vi "helipadDataOrganiser.vi"(3 "Number of Heights":i32=4, 4 "Number of Files":i32=4, 5 "Method A (Left), Method B (Right)":bool, 6 "Data Path":string) -> (0 "Output Data":string[][](array[string]), 1 "Probe No":string, 2 "In Folder":string)   [LabVIEW 2018]
uses:
  <vilib>/Utility/file.llb/Read Delimited Spreadsheet (string).vi
panel:
  in  "Tab Control":enum32{"Pull Method A", "Pull Method B"}(tab)
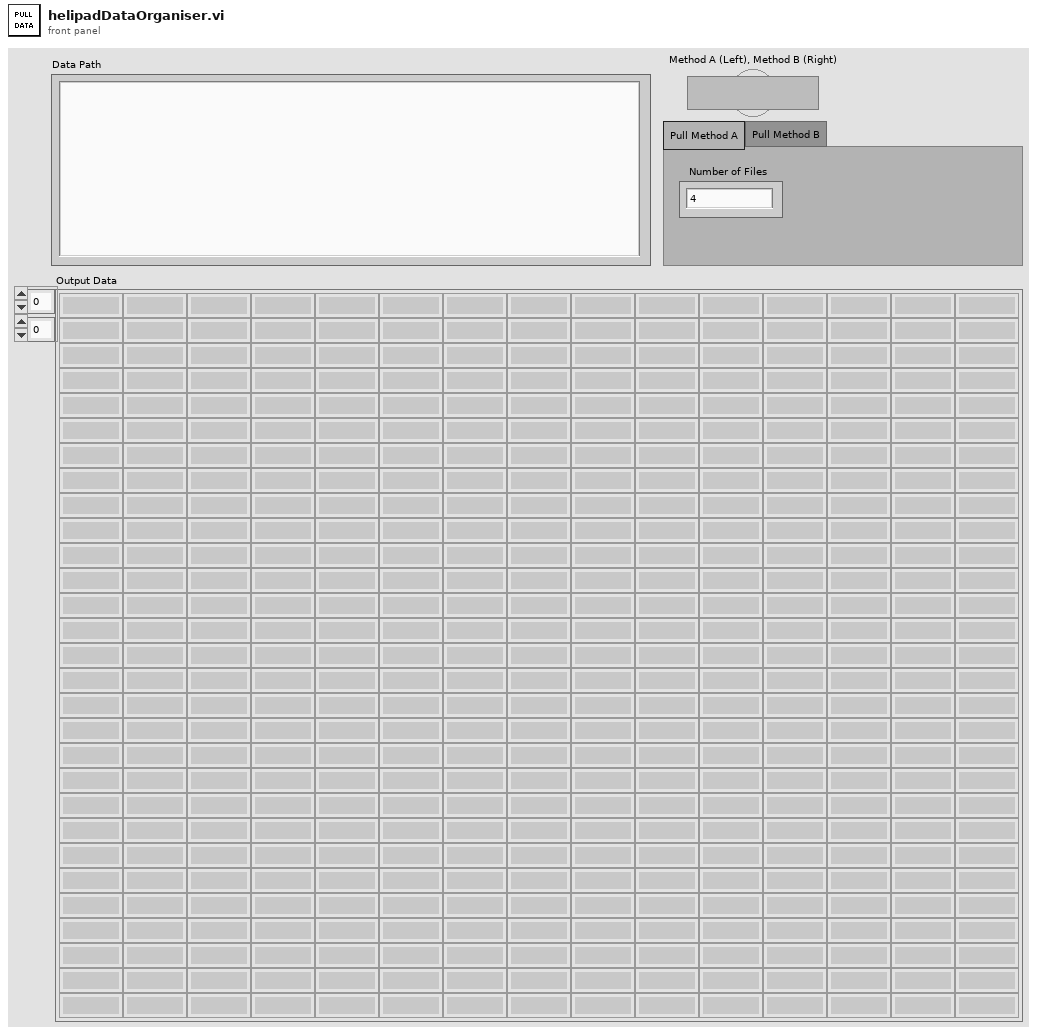
[diagram p1: front panel]
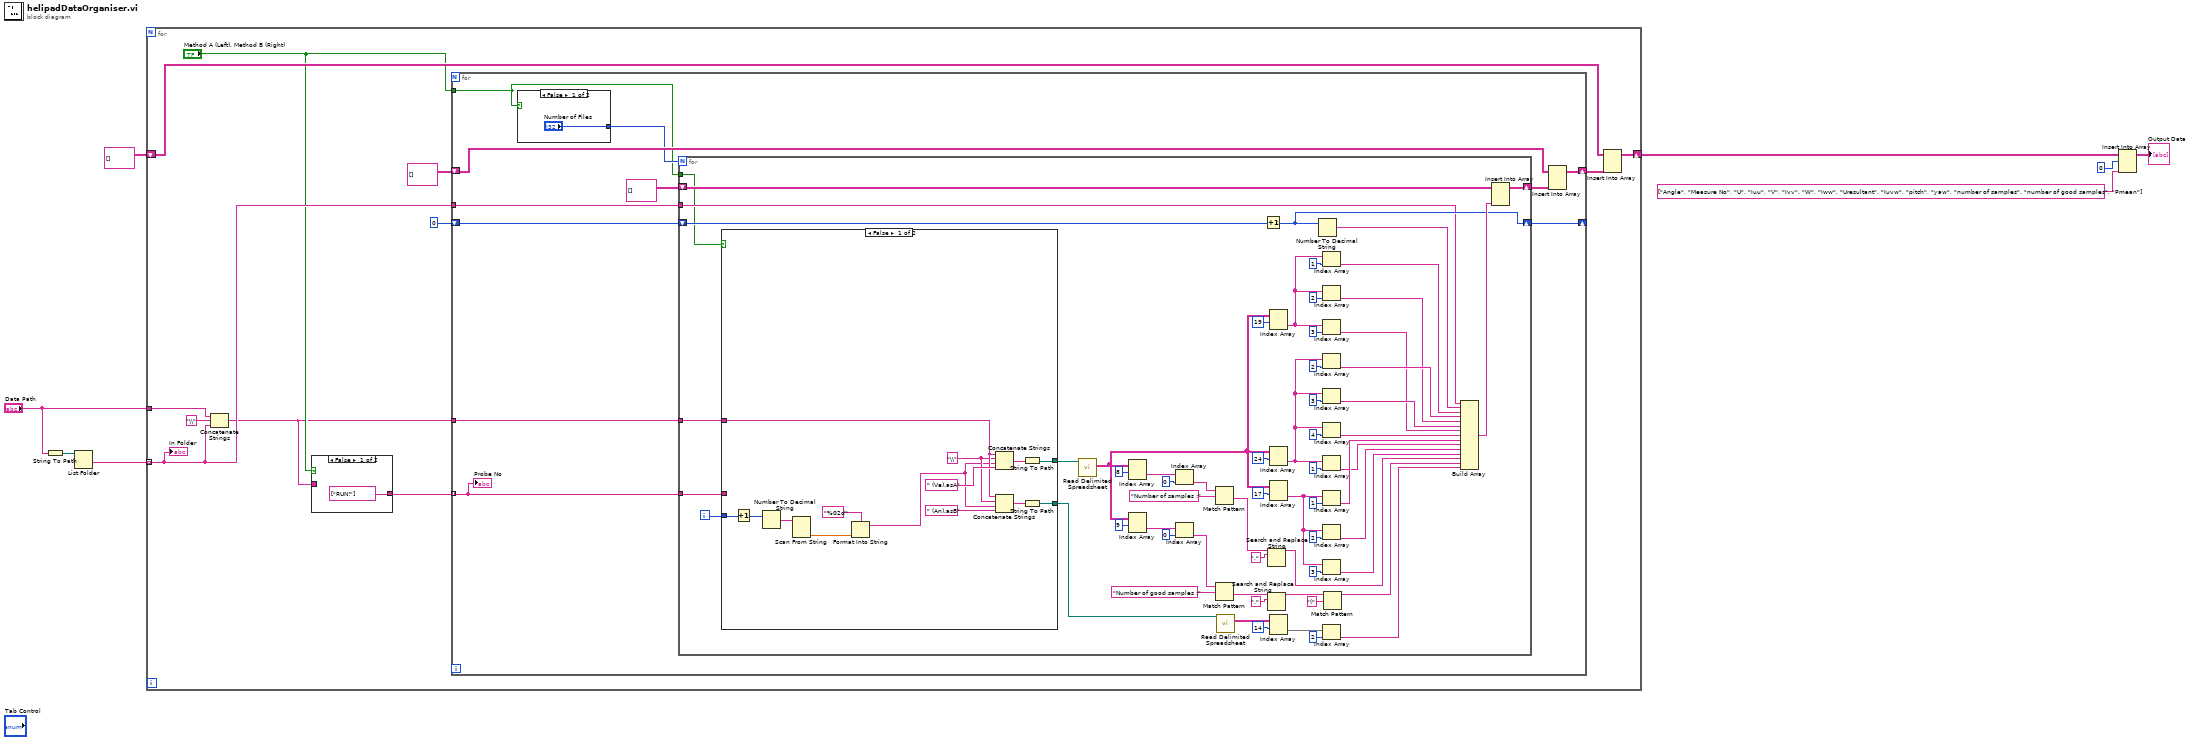
[diagram p0: block diagram]
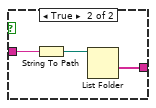
[diagram p2: hidden frame]
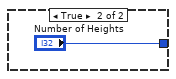
[diagram p3: hidden frame]
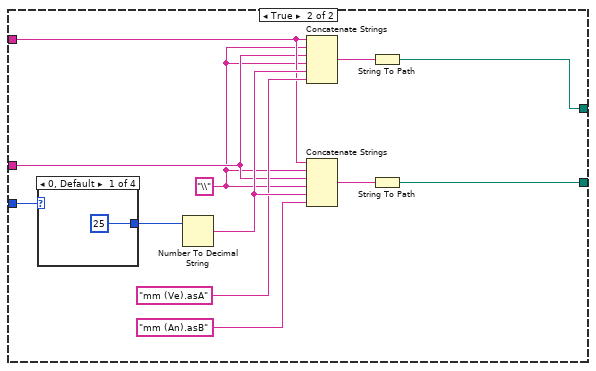
[diagram p4: hidden frame]
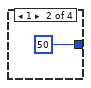
[diagram p5: hidden frame]
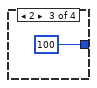
[diagram p6: hidden frame]
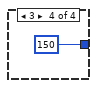
[diagram p7: hidden frame]
diagram:
  n1 = String To Path(string="Data Path") -> (path=w8:path)
  n2 = List Folder(path=w8) -> (folder names=w1:string[])  [unwired: 3 in, 3 out]
  n3 = for {
    shift-right: [w17] -> w6
    shift-left: string[][] [] -> [w13]
    tunnel: w1 -> [w12] mode=indexing
    tunnel: "Data Path" -> [w16]
    n4 = Concatenate Strings(w16, "\\" ("string"), w12) -> (w10:string)
    n5 = case shown="False" "Method A (Left), Method B (Right)" {
      tunnel: w10 -> [_ w22]
      tunnel: [string[] ["RUN!"] ("folder names") w21] -> w9
      frame False {
      }
      frame True {
        n6 = String To Path(string=w22) -> (path=w23:path)
        n7 = List Folder(path=w23) -> (folder names=w21:string[])  [unwired: 3 in, 3 out]
      }
    }
    n8 = for {
      tunnel: w10 -> [w34]
      tunnel: w9 -> [w26] mode=indexing
      shift-right: [w31] -> w14
      shift-left: string[][] [] -> [w30]
      shift-right: [w29] -> _
      shift-left: 0 -> [w28]
      tunnel: w12 -> [w27]
      tunnel: "Method A (Left), Method B (Right)" -> [w24]
      n9 = case shown="False" w24 {
        tunnel: ["Number of Files" "Number of Heights"] -> w25
        frame False {
        }
        frame True {
        }
      }
      n10 = for {
        N: w25 -> [_]
        tunnel: w34 -> [w42]
        tunnel: w26 -> [w41]
        shift-right: [w50] -> w32
        shift-left: string[][] [] -> [w49]
        shift-right: [w44] -> w29
        shift-left: w28 -> [w45]
        tunnel: w27 -> [w43]
        tunnel: w24 -> [w37]
        i -> [w38]
        n11 = case shown="False" w37 {
          tunnel: w42 -> [w111 w119]
          tunnel: w41 -> [_ w118]
          tunnel: [w108 w117] -> w40
          tunnel: [w106 w116] -> w39
          tunnel: w38 -> [w105 w115]
          frame False {
            w110 = "\\" ("string")
            n12 = Increment(x=w105) -> (x+1=w104:i32)
            n13 = Number To Decimal String(number=w104) -> (decimal integer string=w101:string)  [unwired: 1 in]
            n14 = Scan From String(input string=w101) -> (output 1=w102:dbl)  [unwired: 4 in, 3 out]
            n15 = Format Into String(format string="%02d", w102) -> (resulting string=w100:string)  [unwired: 2 in, 1 out]
            n16 = Concatenate Strings(w111, w110, w100, " (Ve).asA" ("string")) -> (w113:string)
            n17 = Concatenate Strings(w111, w110, w100, " (An).asB" ("string")) -> (w107:string)
            n18 = String To Path(string=w113) -> (path=w108:path)
            n19 = String To Path(string=w107) -> (path=w106:path)
          }
          frame True {
            w114 = "\\" ("string")
            n20 = case shown="0, Default" w115 {
              tunnel: [25 50 100 150] -> w122
              frame 0, Default {
              }
              frame 1 {
              }
              frame 2 {
              }
              frame 3 {
              }
            }
            n21 = Number To Decimal String(number=w122) -> (decimal integer string=w125:string)  [unwired: 1 in]
            n22 = Concatenate Strings(w119, w114, w118, w114, w125, "mm (Ve).asA" ("string")) -> (w124:string)
            n23 = Concatenate Strings(w119, w114, w118, w114, w125, "mm (An).asB" ("string")) -> (w123:string)
            n24 = String To Path(string=w124) -> (path=w117:path)
            n25 = String To Path(string=w123) -> (path=w116:path)
          }
        }
        n26 = call-poly <vilib>:"Read Delimited Spreadsheet.vi"("file path (dialog if empty)"=w40) -> ("all rows"=w65:string[][])  [unwired: 9 in, 5 out]
        n27 = Index Array(array=w65, index (row)=8) -> (element=w94:string[])  [unwired: 1 in]
        n28 = Index Array(array=w65, index (row)=9) -> (element=w83:string[])  [unwired: 1 in]
        n29 = Index Array(array=w94, index=0) -> (element=w92:string)
        n30 = Index Array(array=w83, index=0) -> (element=w85:string)
        n31 = Match Pattern(string=w92, regular expression="Number of samples :") -> (after substring=w90:string)  [unwired: 1 in, 3 out]
        n32 = Match Pattern(string=w85, regular expression="Number of good samples :") -> (after substring=w87:string)  [unwired: 1 in, 3 out]
        n33 = call-poly <vilib>:"Read Delimited Spreadsheet.vi"("file path (dialog if empty)"=w39) -> ("all rows"=w99:string[][])  [unwired: 9 in, 5 out]
        n34 = Increment(x=w45) -> (x+1=w44:i32)
        n35 = Search and Replace String(input string=w90, search string=",") -> (result string=w48:string)  [unwired: 6 in, 3 out]
        n36 = Search and Replace String(input string=w87, search string=",") -> (result string=w81:string)  [unwired: 6 in, 3 out]
        n37 = Index Array(array=w65, index (row)=19) -> (element=w73:string[])  [unwired: 1 in]
        n38 = Index Array(array=w65, index (row)=24) -> (element=w58:string[])  [unwired: 1 in]
        n39 = Index Array(array=w65, index (row)=17) -> (element=w76:string[])  [unwired: 1 in]
        n40 = Index Array(array=w99, index (row)=14) -> (element=w97:string[])  [unwired: 1 in]
        n41 = Number To Decimal String(number=w44) -> (decimal integer string=w52:string)  [unwired: 1 in]
        n42 = Index Array(array=w73, index=1) -> (element=w61:string)
        n43 = Index Array(array=w73, index=2) -> (element=w60:string)
        n44 = Index Array(array=w73, index=3) -> (element=w59:string)
        n45 = Index Array(array=w58, index=2) -> (element=w64:string)
        n46 = Index Array(array=w58, index=3) -> (element=w63:string)
        n47 = Index Array(array=w58, index=4) -> (element=w62:string)
        n48 = Index Array(array=w58, index=1) -> (element=w55:string)
        n49 = Index Array(array=w76, index=1) -> (element=w56:string)
        n50 = Index Array(array=w76, index=2) -> (element=w54:string)
        n51 = Index Array(array=w76, index=3) -> (element=w53:string)
        n52 = Index Array(array=w97, index=2) -> (element=w46:string)
        n53 = Match Pattern(string=w81, regular expression="(") -> (before substring=w47:string)  [unwired: 1 in, 3 out]
        n54 = Build Array(w43, w52, w61, w64, w60, w63, w59, w62, w56, w55, w54, w53, w48, w47, w46) -> (w51:string[])
        n55 = Insert Into Array(array=w49, new element=w51) -> (w50:string[][])  [unwired: 2 in]
      }
      n56 = Insert Into Array(array=w30, new element=w32) -> (w31:string[][])  [unwired: 2 in]
      "Probe No" <- w26
    }
    n57 = Insert Into Array(array=w13, new element=w14) -> (w17:string[][])  [unwired: 2 in]
    "In Folder" <- w12
  }
  n58 = Insert Into Array(array=w6, index (row)=0, new element=string[] ["Angle", "Measure No", "U", "Iuu", "V", "Ivv", "W", "Iww", "Uresultant", "Iuvw", "pitch", "yaw", "number of samples", "number of good samples", "Pmean"]) -> (→"Output Data":string[][])  [unwired: 1 in]
